vi "S4GUI_003.vi"(7 "Tab ObsEng":enum32{"Obs", "CCD modes", "Guider", "Eng"}(tab)) -> ()   [LabVIEW 2018] (continued)
        n2644 = call "Write GFOC.vi"("error in (no error)"=w5462, "Opt_Continuous.lvclass"=w5460, "Instrument in"=w5452) -> ("error out"=w5444:errorcluster, "Instrument out"=w5445:refnum<class "Instrument.lvclass">)  [unwired: 7 in]
        n2645 = call "Write Instrument.lvclass.vi"("error in (no error)"=w5444, "Instrument.lvclass"=w5445, "S4ACS_GUI in"=w5524) -> ("error out"=w5443:errorcluster, "S4ACS_GUI out"=w5442:refnum<class "S4GUI.lvclass">)  [unwired: 7 in]
      }
      event "Tab Acq Type": Value Change {
        # "Tab for choosing ACQUISITION MODE: Object, Test, Dflat, Sflat, Dark, Zero, Focus"
        n2646 = event-data() -> ("NewVal"=w5565:T1)  [unwired: 1 in]
        n2647 = case shown="\"ZERO\"" w5565 {
          tunnel: ["OBJECT" "OBJECT" "FLAT" "FLAT" "DARK" "ZERO" "FOCUS"] -> w5542
          tunnel: [w5634 w5639 w5647 w5652 w5657 w5662 w5667] -> w5541
          tunnel: [w5635 w5640 w5646 w5651 w5656 w5661 w5666] -> w5564
          tunnel: [w5636 w5641 w5645 w5650 w5655 w5660 w5665] -> w5538
          tunnel: [u32 0 u32 1 u32 2 u32 3 u32 4 u32 5 u32 6] -> w5533
          frame "OBJECT", Default {
            n2648 = local read "Object_obj"() -> (w5634:string)
            n2649 = local read "OBJECT Comments"() -> (w5636:string)
            n2650 = local read "object suffix"() -> (w5635:string)
          }
          frame "TEST" {
            n2651 = local read "TEST Comments"() -> (w5641:string)
            n2652 = local read "Object_test"() -> (w5639:string)
            n2653 = local read "test suffix"() -> (w5640:string)
          }
          frame "DFLAT" {
            n2654 = local read "DFLAT Comments"() -> (w5645:string)
            n2655 = local read "Object_dflat"() -> (w5647:string)
            n2656 = local read "dflat suffix"() -> (w5646:string)
          }
          frame "SFLAT" {
            n2657 = local read "SFLAT Comments"() -> (w5650:string)
            n2658 = local read "Object_sflat"() -> (w5652:string)
            n2659 = local read "sflat suffix"() -> (w5651:string)
          }
          frame "DARK" {
            n2660 = local read "Object_dark"() -> (w5657:string)
            n2661 = local read "dark suffix"() -> (w5656:string)
            n2662 = local read "DARK Comments"() -> (w5655:string)
          }
          frame "ZERO" {
            n2663 = local read "ZERO Comments"() -> (w5660:string)
            n2664 = local read "Object_zero"() -> (w5662:string)
            n2665 = local read "zero suffix"() -> (w5661:string)
          }
          frame "FOCUS" {
            n2666 = local read "FOCUS Comments"() -> (w5665:string)
            n2667 = local read "Object_focus"() -> (w5667:string)
            n2668 = local read "focus suffix"() -> (w5666:string)
          }
        }
        n2669 = local read "Observer"() -> (w5563:string)
        n2670 = call-dynamic "Write ExpMode.vi"("error in (no error)"=w5566, "ExpMode"=w5565, "S4GUI in"=w5567) -> ("error out"=w5559:errorcluster, "S4GUI out"=w5558:refnum<class "S4GUI.lvclass">)  [unwired: 7 in]
        n2671 = Concatenate Strings("ACQ TAB SELECTED:" ("User Event"), w5542) -> (w5560:string)
        n2672 = call-dynamic "Write User Event.vi"("error in (no error)"=w5559, "User Event"=w5560, "S4GUI in"=w5558) -> ("error out"=w5532:errorcluster, "S4GUI out"=w5531:refnum<class "S4GUI.lvclass">)  [unwired: 7 in]
        n2673 = call-dynamic "Write TabAcqType index.vi"("error in (no error)"=w5532, "TabAcqType index"=w5533, "S4GUI in"=w5531) -> ("error out"=w5528:errorcluster, "S4GUI out"=w5530:refnum<class "S4GUI.lvclass">)  [unwired: 7 in]
        n2674 = call-dynamic "Save TabAcqType index.vi"("error in (no error)"=w5528, "S4GUI in"=w5530) -> ("error out"=w5527:errorcluster, "S4GUI out"=w5529:refnum<class "S4GUI.lvclass">)  [unwired: 8 in]
        n2675 = call-dynamic "Read Publisher.lvclass.vi"("error in (no error)"=w5527, "S4GUI in"=w5529) -> ("error out"=w5556:errorcluster, "Publisher.lvclass"=w5552:refnum<class "Publisher.lvclass">, "S4GUI out"=w5557:refnum<class "S4GUI.lvclass">)  [unwired: 7 in]
        n2676 = call-dynamic "Write object.vi"("error in (no error)"=w5556, "object"=w5541, "Publisher in"=w5552) -> ("error out"=w5555:errorcluster, "Publisher out"=w5551:refnum<class "Publisher.lvclass">)  [unwired: 7 in]
        n2677 = call-dynamic "Write obstype.vi"("error in (no error)"=w5555, "obstype"=w5542, "Publisher in"=w5551) -> ("error out"=w5554:errorcluster, "Publisher out"=w5550:refnum<class "Publisher.lvclass">)  [unwired: 7 in]
        n2678 = call-dynamic "Write observer.vi"("error in (no error)"=w5554, "observer"=w5540, "Publisher in"=w5550) -> ("error out"=w5553:errorcluster, "Publisher out"=w5549:refnum<class "Publisher.lvclass">)  [unwired: 7 in]
        n2679 = call-dynamic "Write projid.vi"("error in (no error)"=w5553, "projid"=w5539, "Publisher in"=w5549) -> ("error out"=w5546:errorcluster, "Publisher out"=w5545:refnum<class "Publisher.lvclass">)  [unwired: 7 in]
        n2680 = call-dynamic "Write comments.vi"("error in (no error)"=w5546, "comments"=w5538, "Publisher in"=w5545) -> ("error out"=w5548:errorcluster, "Publisher out"=w5547:refnum<class "Publisher.lvclass">)  [unwired: 7 in]
        n2681 = call-dynamic "Write Publisher.lvclass.vi"("error in (no error)"=w5548, "Publisher.lvclass"=w5547, "S4GUI in"=w5557) -> ("error out"=w5544:errorcluster, "S4GUI out"=w5543:refnum<class "S4GUI.lvclass">)  [unwired: 7 in]
        n2682 = call-dynamic "Read AcquisitionA.vi"("error in (no error)"=w5544, "S4ACS_GUI in"=w5543) -> ("error out"=w5574:errorcluster, "Acquisition.lvclass"=w5575:refnum<class "Acquisition.lvclass">, "S4ACS_GUI out"=w5594:refnum<class "S4GUI.lvclass">)  [unwired: 7 in]
        n2683 = call-dynamic "Read AcquisitionC.vi"("error in (no error)"=w5532, "S4ACS_GUI in"=w5531) -> ("error out"=w5570:errorcluster, "Acquisition.lvclass"=w5571:refnum<class "Acquisition.lvclass">)  [unwired: 7 in, 1 out]
        n2684 = call "Read AcquisitionB.vi"("error in (no error)"=w5532, "S4ACS_GUI in"=w5531) -> ("error out"=w5572:errorcluster, "Acquisition.lvclass"=w5573:refnum<class "Acquisition.lvclass">)  [unwired: 7 in, 1 out]
        n2685 = call-dynamic "Read AcquisitionD.vi"("error in (no error)"=w5532, "S4ACS_GUI in"=w5531) -> ("error out"=w5568:errorcluster, "Acquisition.lvclass"=w5569:refnum<class "Acquisition.lvclass">)  [unwired: 7 in, 1 out]
        n2686 = To Lower Case(string=w5564) -> (all lower case string=w5562:string)
        n2687 = case shown="\"ZERO\"" w5565 {
          tunnel: [w5902 w6271 w6680] -> w5593
          tunnel: [w5901 w6270 w6679] -> w5592
          tunnel: [w5900 w6269 w6678] -> w5590
          tunnel: [w5899 w6268 w6677] -> w5589
          tunnel: [w5898 w6267 w6676] -> w5579
          tunnel: [w5897 w6266 w6675] -> w5578
          tunnel: [w5896 w6265 w6674] -> w5577
          tunnel: [w5895 w6264 w6673] -> w5576
          tunnel: w5575 -> [w5894 w6263 w6672]
          tunnel: w5574 -> [w5893 w6262 w6671]
          tunnel: w5573 -> [w5883 w6253 w6662]
          tunnel: w5572 -> [w5882 w6252 w6661]
          tunnel: w5571 -> [w5881 w6251 w6660]
          tunnel: w5570 -> [w5880 w6250 w6659]
          tunnel: w5569 -> [w5879 w6249 w6658]
          tunnel: w5568 -> [w5878 w6248 w6657]
          tunnel: w5541 -> [w5875 w6247 w6656]
          tunnel: w5538 -> [w5876 w6246 w6655]
          tunnel: w5563 -> [w5877 w6245 w6654]
          tunnel: w5562 -> [w5874 w6244 w6653]
          tunnel: w5542 -> [w5873 w6243 w6652]
          frame "ZERO" {
            w5892 = 1e-05 ("Exptime ch1")
            # "nome do arquivo .cfg"
            # "seção no arquivo .cfg"
            # "nome do arquivo .cfg"
            # "seção no arquivo .cfg"
            # "nome do arquivo .cfg"
            # "seção no arquivo .cfg"
            # "nome do arquivo .cfg"
            # "seção no arquivo .cfg"
            # "ZERO: EXPTIME=1E-5 (mandatory), shutter automatically closed, save current FRAME_TRANSFER (prev_FT) and reset FRAME_TRANSFER."
            n2688 = call "Read connection.vi"("error in (no error)"=w5880, "Server in"=w5881) -> ("error out"=w5886:errorcluster, "connection"=w5720:bool, "Server out"=w5887:refnum<class "Acquisition.lvclass">)  [unwired: 7 in]
            n2689 = call "Read connection.vi"("error in (no error)"=w5882, "Server in"=w5883) -> ("error out"=w5888:errorcluster, "connection"=w5771:bool, "Server out"=w5889:refnum<class "Acquisition.lvclass">)  [unwired: 7 in]
            n2690 = call "Read connection.vi"("error in (no error)"=w5893, "Server in"=w5894) -> ("error out"=w5890:errorcluster, "connection"=w5822:bool, "Server out"=w5891:refnum<class "Acquisition.lvclass">)  [unwired: 7 in]
            n2691 = call "Read connection.vi"("error in (no error)"=w5878, "Server in"=w5879) -> ("error out"=w5884:errorcluster, "connection"=w5669:bool, "Server out"=w5885:refnum<class "Acquisition.lvclass">)  [unwired: 7 in]
            n2692 = call-dynamic "Read Channel.vi"("error in (no error)"=w5888, "Acquisition in"=w5889) -> ("error out"=w5809:errorcluster, "Channel.lvclass"=w5808:refnum<class "Channel.lvclass">, "Acquisition out"=w5807:refnum<class "Acquisition.lvclass">)  [unwired: 7 in]
            n2693 = call-dynamic "Read Channel.vi"("error in (no error)"=w5884, "Acquisition in"=w5885) -> ("error out"=w5717:errorcluster, "Channel.lvclass"=w5718:refnum<class "Channel.lvclass">, "Acquisition out"=w5719:refnum<class "Acquisition.lvclass">)  [unwired: 7 in]
            n2694 = call-dynamic "Read Channel.vi"("error in (no error)"=w5886, "Acquisition in"=w5887) -> ("error out"=w5758:errorcluster, "Channel.lvclass"=w5757:refnum<class "Channel.lvclass">, "Acquisition out"=w5756:refnum<class "Acquisition.lvclass">)  [unwired: 7 in]
            n2695 = call-dynamic "Read Channel.vi"("error in (no error)"=w5890, "Acquisition in"=w5891) -> ("error out"=w5870:errorcluster, "Channel.lvclass"=w5871:refnum<class "Channel.lvclass">, "Acquisition out"=w5872:refnum<class "Acquisition.lvclass">)  [unwired: 7 in]
            n2696 = call-dynamic "Read Interface.vi"("error in (no error)"=w5717, "Channel in"=w5718) -> ("error out"=w5683:errorcluster, "Interface.lvclass"=w5682:refnum<class "Interface.lvclass">, "Channel out"=w5679:refnum<class "Channel.lvclass">)  [unwired: 7 in]
            n2697 = call-dynamic "Read Interface.vi"("error in (no error)"=w5809, "Channel in"=w5808) -> ("error out"=w5783:errorcluster, "Interface.lvclass"=w5784:refnum<class "Interface.lvclass">, "Channel out"=w5778:refnum<class "Channel.lvclass">)  [unwired: 7 in]
            n2698 = call-dynamic "Read Interface.vi"("error in (no error)"=w5758, "Channel in"=w5757) -> ("error out"=w5732:errorcluster, "Interface.lvclass"=w5733:refnum<class "Interface.lvclass">, "Channel out"=w5730:refnum<class "Channel.lvclass">)  [unwired: 7 in]
            n2699 = call-dynamic "Read Interface.vi"("error in (no error)"=w5870, "Channel in"=w5871) -> ("error out"=w5839:errorcluster, "Interface.lvclass"=w5840:refnum<class "Interface.lvclass">, "Channel out"=w5833:refnum<class "Channel.lvclass">)  [unwired: 7 in]
            n2700 = call-dynamic "Write restoreExpTime.vi"("error in (no error)"=w5683, "restoreExpTime"=TRUE, "Interface in"=w5682) -> ("error out"=w5676:errorcluster, "Interface out"=w5681:refnum<class "Interface.lvclass">)  [unwired: 7 in]
            n2701 = call-dynamic "Write restoreExpTime.vi"("error in (no error)"=w5783, "restoreExpTime"=TRUE, "Interface in"=w5784) -> ("error out"=w5780:errorcluster, "Interface out"=w5782:refnum<class "Interface.lvclass">)  [unwired: 7 in]
            n2702 = call-dynamic "Write restoreExpTime.vi"("error in (no error)"=w5732, "restoreExpTime"=TRUE, "Interface in"=w5733) -> ("error out"=w5725:errorcluster, "Interface out"=w5731:refnum<class "Interface.lvclass">)  [unwired: 7 in]
            n2703 = call-dynamic "Write restoreExpTime.vi"("error in (no error)"=w5839, "restoreExpTime"=TRUE, "Interface in"=w5840) -> ("error out"=w5829:errorcluster, "Interface out"=w5830:refnum<class "Interface.lvclass">)  [unwired: 7 in]
            n2704 = property on="Exptime ch1" class="DigNum (strict)"("Value"=w5892) -> ()  [unwired: 2 in, 2 out]
            n2705 = call-dynamic "Read target cluster.vi"("error in (no error)"=w5780, "Channel in"=w5778) -> ("error out"=w5779:errorcluster, "target cluster"=w5781:T31, "Channel out"=w5774:refnum<class "Channel.lvclass">)  [unwired: 7 in]
            n2706 = stacked-sequence {
              tunnel: [_ w5994] -> w5777
              tunnel: w5781 -> [_ w5993]
              tunnel: w5781 -> [w5991 _]
              tunnel: [w5990 _] -> w5786
              frame #0 {
                n2707 = Unbundle By Name(w5991) -> ("FRAME_TRANSFER"=w5990:bool)
              }
              frame #1 {
                # "closed"
                n2708 = Bundle By Name(cluster=w5993, "SHUTTER_MODE"=u8 2, "FRAME_TRANSFER"=FALSE) -> (w5994:T31)
              }
            }
            n2709 = call-dynamic "Read target cluster.vi"("error in (no error)"=w5676, "Channel in"=w5679) -> ("error out"=w5675:errorcluster, "target cluster"=w5677:T31, "Channel out"=w5678:refnum<class "Channel.lvclass">)  [unwired: 7 in]
            n2710 = stacked-sequence {
              tunnel: w5677 -> [_ w5933]
              tunnel: [_ w5932] -> w5673
              tunnel: w5677 -> [w5929 _]
              tunnel: [w5928 _] -> w5685
              frame #0 {
                n2711 = Unbundle By Name(w5929) -> ("FRAME_TRANSFER"=w5928:bool)
              }
              frame #1 {
                # "closed"
                n2712 = Bundle By Name(cluster=w5933, "SHUTTER_MODE"=u8 2, "FRAME_TRANSFER"=FALSE) -> (w5932:T31)
              }
            }
            n2713 = call-dynamic "Read target cluster.vi"("error in (no error)"=w5725, "Channel in"=w5730) -> ("error out"=w5724:errorcluster, "target cluster"=w5726:T31, "Channel out"=w5722:refnum<class "Channel.lvclass">)  [unwired: 7 in]
            n2714 = stacked-sequence {
              tunnel: [_ w5963] -> w5728
              tunnel: w5726 -> [_ w5962]
              tunnel: w5726 -> [w5960 _]
              tunnel: [w5959 _] -> w5735
              frame #0 {
                n2715 = Unbundle By Name(w5960) -> ("FRAME_TRANSFER"=w5959:bool)
              }
              frame #1 {
                # "closed"
                n2716 = Bundle By Name(cluster=w5962, "SHUTTER_MODE"=u8 2, "FRAME_TRANSFER"=FALSE) -> (w5963:T31)
              }
            }
            n2717 = property on="Exptime ch2" class="DigNum (strict)"("Value"=w5892) -> ()  [unwired: 2 in, 2 out]
            n2718 = call-dynamic "Read target cluster.vi"("error in (no error)"=w5829, "Channel in"=w5833) -> ("error out"=w5828:errorcluster, "target cluster"=w5831:T31, "Channel out"=w5832:refnum<class "Channel.lvclass">)  [unwired: 7 in]
            n2719 = stacked-sequence {
              tunnel: [_ w6026] -> w5837
              tunnel: w5831 -> [_ w6023]
              tunnel: w5831 -> [w6022 _]
              tunnel: [w6021 _] -> w5841
              frame #0 {
                n2720 = Unbundle By Name(w6022) -> ("FRAME_TRANSFER"=w6021:bool)
              }
              frame #1 {
                # "closed"
                n2721 = Bundle By Name(cluster=w6023, "SHUTTER_MODE"=u8 2, "FRAME_TRANSFER"=FALSE) -> (w6026:T31)
              }
            }
            n2722 = call-dynamic "Write PREV_FT.vi"("error in (no error)"=w5779, "PREV_FT"=w5786, "Interface in"=w5782) -> ("error out"=w5776:errorcluster, "Interface out"=w5772:refnum<class "Interface.lvclass">)  [unwired: 7 in]
            n2723 = call-dynamic "Write PREV_FT.vi"("error in (no error)"=w5675, "PREV_FT"=w5685, "Interface in"=w5681) -> ("error out"=w5674:errorcluster, "Interface out"=w5680:refnum<class "Interface.lvclass">)  [unwired: 7 in]
            n2724 = call-dynamic "Write PREV_FT.vi"("error in (no error)"=w5724, "PREV_FT"=w5735, "Interface in"=w5731) -> ("error out"=w5727:errorcluster, "Interface out"=w5729:refnum<class "Interface.lvclass">)  [unwired: 7 in]
            n2725 = property on="Exptime ch3" class="DigNum (strict)"("Value"=w5892) -> ()  [unwired: 2 in, 2 out]
            n2726 = call-dynamic "Write PREV_FT.vi"("error in (no error)"=w5828, "PREV_FT"=w5841, "Interface in"=w5830) -> ("error out"=w5834:errorcluster, "Interface out"=w5827:refnum<class "Interface.lvclass">)  [unwired: 7 in]
            n2727 = call-dynamic "Write target cluster.vi"("error in (no error)"=w5776, "target cluster"=w5777, "Channel in"=w5774) -> ("error out"=w5775:errorcluster, "Channel out"=w5773:refnum<class "Channel.lvclass">)  [unwired: 7 in]
            n2728 = call-dynamic "Write target cluster.vi"("error in (no error)"=w5674, "target cluster"=w5673, "Channel in"=w5678) -> ("error out"=w5672:errorcluster, "Channel out"=w5671:refnum<class "Channel.lvclass">)  [unwired: 7 in]
            n2729 = call-dynamic "Write target cluster.vi"("error in (no error)"=w5727, "target cluster"=w5728, "Channel in"=w5722) -> ("error out"=w5723:errorcluster, "Channel out"=w5721:refnum<class "Channel.lvclass">)  [unwired: 7 in]
            n2730 = call-dynamic "Write target cluster.vi"("error in (no error)"=w5834, "target cluster"=w5837, "Channel in"=w5832) -> ("error out"=w5836:errorcluster, "Channel out"=w5835:refnum<class "Channel.lvclass">)  [unwired: 7 in]
            n2731 = Flatten To String(anything=w5777, error in (no error)=w5775) -> (data string=w5810:string, error out=w5811:errorcluster)  [unwired: 2 in, 1 out]
            n2732 = Flatten To String(anything=w5673, error in (no error)=w5672) -> (data string=w5716:string, error out=w5715:errorcluster)  [unwired: 2 in, 1 out]
            n2733 = Flatten To String(anything=w5728, error in (no error)=w5723) -> (data string=w5759:string, error out=w5760:errorcluster)  [unwired: 2 in, 1 out]
            n2734 = Flatten To String(anything=w5837, error in (no error)=w5836) -> (data string=w5869:string, error out=w5868:errorcluster)  [unwired: 2 in, 1 out]
            n2735 = property on="Exptime ch4" class="DigNum (strict)"("Value"=w5892) -> ()  [unwired: 2 in, 2 out]
            n2736 = call "Write flatted cluster.vi"("error in (no error)"=w5811, "flatted cluster"=w5810, "Interface in"=w5772) -> ("error out"=w5813:errorcluster, "Interface out"=w5812:refnum<class "Interface.lvclass">)  [unwired: 7 in]
            n2737 = call "Write flatted cluster.vi"("error in (no error)"=w5715, "flatted cluster"=w5716, "Interface in"=w5680) -> ("error out"=w5713:errorcluster, "Interface out"=w5714:refnum<class "Interface.lvclass">)  [unwired: 7 in]
            n2738 = call "Write flatted cluster.vi"("error in (no error)"=w5760, "flatted cluster"=w5759, "Interface in"=w5729) -> ("error out"=w5762:errorcluster, "Interface out"=w5761:refnum<class "Interface.lvclass">)  [unwired: 7 in]
            n2739 = call "Write flatted cluster.vi"("error in (no error)"=w5868, "flatted cluster"=w5869, "Interface in"=w5827) -> ("error out"=w5866:errorcluster, "Interface out"=w5867:refnum<class "Interface.lvclass">)  [unwired: 7 in]
            n2740 = call-dynamic "Write Interface.vi"("error in (no error)"=w5813, "Interface.lvclass"=w5812, "Channel in"=w5773) -> ("error out"=w5815:errorcluster, "Channel out"=w5816:refnum<class "Channel.lvclass">)  [unwired: 7 in]
            n2741 = call-dynamic "Write Interface.vi"("error in (no error)"=w5713, "Interface.lvclass"=w5714, "Channel in"=w5671) -> ("error out"=w5711:errorcluster, "Channel out"=w5710:refnum<class "Channel.lvclass">)  [unwired: 7 in]
            n2742 = call-dynamic "Write Interface.vi"("error in (no error)"=w5762, "Interface.lvclass"=w5761, "Channel in"=w5721) -> ("error out"=w5764:errorcluster, "Channel out"=w5765:refnum<class "Channel.lvclass">)  [unwired: 7 in]
            n2743 = call-dynamic "Write Interface.vi"("error in (no error)"=w5866, "Interface.lvclass"=w5867, "Channel in"=w5835) -> ("error out"=w5864:errorcluster, "Channel out"=w5863:refnum<class "Channel.lvclass">)  [unwired: 7 in]
            n2744 = call "Write section_name.vi"("error in (no error)"=w5815, "section_name"="CCD_ACS2", "Channel in"=w5816) -> ("error out"=w5814:errorcluster, "Channel out"=w5819:refnum<class "Channel.lvclass">)  [unwired: 7 in]
            n2745 = call "Write section_name.vi"("error in (no error)"=w5711, "section_name"="CCD_ACS4", "Channel in"=w5710) -> ("error out"=w5712:errorcluster, "Channel out"=w5707:refnum<class "Channel.lvclass">)  [unwired: 7 in]
            n2746 = call "Write section_name.vi"("error in (no error)"=w5764, "section_name"="CCD_ACS3", "Channel in"=w5765) -> ("error out"=w5763:errorcluster, "Channel out"=w5768:refnum<class "Channel.lvclass">)  [unwired: 7 in]
            n2747 = call "Write section_name.vi"("error in (no error)"=w5864, "section_name"="CCD_ACS1", "Channel in"=w5863) -> ("error out"=w5865:errorcluster, "Channel out"=w5860:refnum<class "Channel.lvclass">)  [unwired: 7 in]
            n2748 = call-dynamic "save config.vi"("error in (no error)"=w5814, "file config"="lastsaved.cfg", "Channel in"=w5819) -> ("error out"=w5789:errorcluster, "Channel out"=w5790:refnum<class "Channel.lvclass">)  [unwired: 7 in]
            n2749 = call-dynamic "save config.vi"("error in (no error)"=w5712, "file config"="lastsaved.cfg", "Channel in"=w5707) -> ("error out"=w5688:errorcluster, "Channel out"=w5689:refnum<class "Channel.lvclass">)  [unwired: 7 in]
            n2750 = call-dynamic "save config.vi"("error in (no error)"=w5763, "file config"="lastsaved.cfg", "Channel in"=w5768) -> ("error out"=w5737:errorcluster, "Channel out"=w5739:refnum<class "Channel.lvclass">)  [unwired: 7 in]
            n2751 = call-dynamic "save config.vi"("error in (no error)"=w5865, "file config"="lastsaved.cfg", "Channel in"=w5860) -> ("error out"=w5850:errorcluster, "Channel out"=w5851:refnum<class "Channel.lvclass">)  [unwired: 7 in]
            n2752 = local read "Filter2"() -> (w5791:u8)
            n2753 = local read "Filter4"() -> (w5705:u8)
            n2754 = local read "Filter3"() -> (w5755:u8)
            n2755 = local read "Filter1"() -> (w5852:u8)
            n2756 = call-dynamic "Write Filter.vi"("error in (no error)"=w5789, "Filter"=w5791, "Channel in"=w5790) -> ("error out"=w5798:errorcluster, "Channel out"=w5799:refnum<class "Channel.lvclass">)  [unwired: 7 in]
            n2757 = call-dynamic "Write Filter.vi"("error in (no error)"=w5688, "Filter"=w5705, "Channel in"=w5689) -> ("error out"=w5698:errorcluster, "Channel out"=w5697:refnum<class "Channel.lvclass">)  [unwired: 7 in]
            n2758 = call-dynamic "Write Filter.vi"("error in (no error)"=w5737, "Filter"=w5755, "Channel in"=w5739) -> ("error out"=w5748:errorcluster, "Channel out"=w5747:refnum<class "Channel.lvclass">)  [unwired: 7 in]
            n2759 = call-dynamic "Write Filter.vi"("error in (no error)"=w5850, "Filter"=w5852, "Channel in"=w5851) -> ("error out"=w5859:errorcluster, "Channel out"=w5849:refnum<class "Channel.lvclass">)  [unwired: 7 in]
            n2760 = call-dynamic "Read Interface.vi"("error in (no error)"=w5798, "Channel in"=w5799) -> ("error out"=w5796:errorcluster, "Interface.lvclass"=w5801:refnum<class "Interface.lvclass">, "Channel out"=w5800:refnum<class "Channel.lvclass">)  [unwired: 7 in]
            n2761 = call-dynamic "Read Interface.vi"("error in (no error)"=w5698, "Channel in"=w5697) -> ("error out"=w5700:errorcluster, "Interface.lvclass"=w5695:refnum<class "Interface.lvclass">, "Channel out"=w5696:refnum<class "Channel.lvclass">)  [unwired: 7 in]
            n2762 = call-dynamic "Read Interface.vi"("error in (no error)"=w5748, "Channel in"=w5747) -> ("error out"=w5750:errorcluster, "Interface.lvclass"=w5745:refnum<class "Interface.lvclass">, "Channel out"=w5746:refnum<class "Channel.lvclass">)  [unwired: 7 in]
            n2763 = call-dynamic "Read Interface.vi"("error in (no error)"=w5859, "Channel in"=w5849) -> ("error out"=w5857:errorcluster, "Interface.lvclass"=w5848:refnum<class "Interface.lvclass">, "Channel out"=w5842:refnum<class "Channel.lvclass">)  [unwired: 7 in]
            n2764 = call-dynamic "Write Suffix.vi"("error in (no error)"=w5796, "Suffix"=w5874, "Interface in"=w5801) -> ("error out"=w5792:errorcluster, "Interface out"=w5802:refnum<class "Interface.lvclass">)  [unwired: 7 in]
            n2765 = call-dynamic "Write Suffix.vi"("error in (no error)"=w5700, "Suffix"=w5874, "Interface in"=w5695) -> ("error out"=w5704:errorcluster, "Interface out"=w5694:refnum<class "Interface.lvclass">)  [unwired: 7 in]
            n2766 = call-dynamic "Write Suffix.vi"("error in (no error)"=w5750, "Suffix"=w5874, "Interface in"=w5745) -> ("error out"=w5754:errorcluster, "Interface out"=w5744:refnum<class "Interface.lvclass">)  [unwired: 7 in]
            n2767 = call-dynamic "Write Suffix.vi"("error in (no error)"=w5857, "Suffix"=w5874, "Interface in"=w5848) -> ("error out"=w5853:errorcluster, "Interface out"=w5847:refnum<class "Interface.lvclass">)  [unwired: 7 in]
            n2768 = call-dynamic "Write ObsType.vi"("error in (no error)"=w5792, "ObsType"=w5873, "Interface in"=w5802) -> ("error out"=w5793:errorcluster, "Interface out"=w5803:refnum<class "Interface.lvclass">)  [unwired: 7 in]
            n2769 = call-dynamic "Write ObsType.vi"("error in (no error)"=w5704, "ObsType"=w5873, "Interface in"=w5694) -> ("error out"=w5703:errorcluster, "Interface out"=w5693:refnum<class "Interface.lvclass">)  [unwired: 7 in]
            n2770 = call-dynamic "Write ObsType.vi"("error in (no error)"=w5754, "ObsType"=w5873, "Interface in"=w5744) -> ("error out"=w5753:errorcluster, "Interface out"=w5743:refnum<class "Interface.lvclass">)  [unwired: 7 in]
            n2771 = call-dynamic "Write ObsType.vi"("error in (no error)"=w5853, "ObsType"=w5873, "Interface in"=w5847) -> ("error out"=w5854:errorcluster, "Interface out"=w5846:refnum<class "Interface.lvclass">)  [unwired: 7 in]
            n2772 = call-dynamic "Write Object.vi"("error in (no error)"=w5793, "Object"=w5875, "Interface in"=w5803) -> ("error out"=w5794:errorcluster, "Interface out"=w5804:refnum<class "Interface.lvclass">)  [unwired: 7 in]
            n2773 = call-dynamic "Write Object.vi"("error in (no error)"=w5703, "Object"=w5875, "Interface in"=w5693) -> ("error out"=w5702:errorcluster, "Interface out"=w5692:refnum<class "Interface.lvclass">)  [unwired: 7 in]
            n2774 = call-dynamic "Write Object.vi"("error in (no error)"=w5753, "Object"=w5875, "Interface in"=w5743) -> ("error out"=w5752:errorcluster, "Interface out"=w5742:refnum<class "Interface.lvclass">)  [unwired: 7 in]
            n2775 = call-dynamic "Write Object.vi"("error in (no error)"=w5854, "Object"=w5875, "Interface in"=w5846) -> ("error out"=w5855:errorcluster, "Interface out"=w5845:refnum<class "Interface.lvclass">)  [unwired: 7 in]
            n2776 = call-dynamic "Write Comments.vi"("error in (no error)"=w5794, "Comments"=w5876, "Interface in"=w5804) -> ("error out"=w5795:errorcluster, "Interface out"=w5805:refnum<class "Interface.lvclass">)  [unwired: 7 in]
            n2777 = call-dynamic "Write Comments.vi"("error in (no error)"=w5702, "Comments"=w5876, "Interface in"=w5692) -> ("error out"=w5701:errorcluster, "Interface out"=w5691:refnum<class "Interface.lvclass">)  [unwired: 7 in]
            n2778 = call-dynamic "Write Comments.vi"("error in (no error)"=w5752, "Comments"=w5876, "Interface in"=w5742) -> ("error out"=w5751:errorcluster, "Interface out"=w5741:refnum<class "Interface.lvclass">)  [unwired: 7 in]
            n2779 = call-dynamic "Write Comments.vi"("error in (no error)"=w5855, "Comments"=w5876, "Interface in"=w5845) -> ("error out"=w5856:errorcluster, "Interface out"=w5844:refnum<class "Interface.lvclass">)  [unwired: 7 in]
            n2780 = call-dynamic "Write Observer.vi"("error in (no error)"=w5701, "Observer"=w5877, "Interface in"=w5691) -> ("error out"=w5699:errorcluster, "Interface out"=w5690:refnum<class "Interface.lvclass">)  [unwired: 7 in]
            n2781 = call-dynamic "Write Observer.vi"("error in (no error)"=w5751, "Observer"=w5877, "Interface in"=w5741) -> ("error out"=w5749:errorcluster, "Interface out"=w5740:refnum<class "Interface.lvclass">)  [unwired: 7 in]
            n2782 = call-dynamic "Write Observer.vi"("error in (no error)"=w5795, "Observer"=w5877, "Interface in"=w5805) -> ("error out"=w5797:errorcluster, "Interface out"=w5806:refnum<class "Interface.lvclass">)  [unwired: 7 in]
            n2783 = call-dynamic "Write Observer.vi"("error in (no error)"=w5856, "Observer"=w5877, "Interface in"=w5844) -> ("error out"=w5858:errorcluster, "Interface out"=w5843:refnum<class "Interface.lvclass">)  [unwired: 7 in]
            n2784 = call-dynamic "Write Interface.vi"("error in (no error)"=w5699, "Interface.lvclass"=w5690, "Channel in"=w5696) -> ("error out"=w5687:errorcluster, "Channel out"=w5686:refnum<class "Channel.lvclass">)  [unwired: 7 in]
            n2785 = call-dynamic "Write Interface.vi"("error in (no error)"=w5749, "Interface.lvclass"=w5740, "Channel in"=w5746) -> ("error out"=w5736:errorcluster, "Channel out"=w5738:refnum<class "Channel.lvclass">)  [unwired: 7 in]
            n2786 = call-dynamic "Write Interface.vi"("error in (no error)"=w5858, "Interface.lvclass"=w5843, "Channel in"=w5842) -> ("error out"=w5825:errorcluster, "Channel out"=w5826:refnum<class "Channel.lvclass">)  [unwired: 7 in]
            n2787 = call-dynamic "Write Interface.vi"("error in (no error)"=w5797, "Interface.lvclass"=w5806, "Channel in"=w5800) -> ("error out"=w5788:errorcluster, "Channel out"=w5787:refnum<class "Channel.lvclass">)  [unwired: 7 in]
            n2788 = case shown="True" w5822 {
              tunnel: w5826 -> [w5997 w6001]
              tunnel: w5825 -> [w5996 w6000]
              tunnel: [w5997 w5999] -> w5824
              tunnel: [w5996 w5998] -> w5823
              frame False {
              }
              frame True {
                n2789 = call-dynamic "Read State Machine.vi"("error in (no error)"=w6000, "Device in"=w6001) -> ("error out"=w6003:errorcluster, "State Machine.lvclass"=w6006:refnum<class "State Machine.lvclass">, "Device out"=w6018:refnum<class "Channel.lvclass">)  [unwired: 7 in]
                n2790 = call-dynamic "Read ref StatesQueue.vi"("error in (no error)"=w6003, "State Machine in"=w6006) -> ("error out"=w6010:errorcluster, "ref StatesQueue"=w6009:refnum<queue>, "State Machine out"=w6005:refnum<class "State Machine.lvclass">)  [unwired: 7 in]
                n2791 = Flush Queue(queue=w6009, error in (no error)=w6010) -> (queue out=w6011:refnum<queue>, error out=w6015:errorcluster)  [unwired: 1 out]
                n2792 = Enqueue Element(queue=w6011, element=u32 300 ("State"), error in (no error)=w6015) -> (queue out=w6012:refnum<queue>, error out=w6016:errorcluster)  [unwired: 1 in, 1 out]
                n2793 = Enqueue Element(queue=w6012, element=u32 60 ("State"), error in (no error)=w6016) -> (queue out=w6013:refnum<queue>, error out=w6014:errorcluster)  [unwired: 1 in, 1 out]
                n2794 = call-dynamic "Write ref StatesQueue.vi"("error in (no error)"=w6014, "ref StatesQueue"=w6013, "State Machine in"=w6005) -> ("error out"=w6002:errorcluster, "State Machine out"=w6004:refnum<class "State Machine.lvclass">)  [unwired: 7 in]
                n2795 = call-dynamic "Write State.vi"("error in (no error)"=w6002, "State"=0, "State Machine in"=w6004) -> ("error out"=w6020:errorcluster, "State Machine out"=w6017:refnum<class "State Machine.lvclass">)  [unwired: 7 in]
                n2796 = call-dynamic "Write State Machine.vi"("error in (no error)"=w6020, "State Machine.lvclass"=w6017, "Device in"=w6018) -> ("error out"=w5998:errorcluster, "Device out"=w5999:refnum<class "Channel.lvclass">)  [unwired: 7 in]
              }
            }
            n2797 = case shown="True" w5771 {
              tunnel: [w5965 w5989] -> w5821
              tunnel: [w5966 w5988] -> w5820
              tunnel: w5788 -> [w5965 w5983]
              tunnel: w5787 -> [w5966 w5982]
              frame False {
              }
              frame True {
                n2798 = call-dynamic "Read State Machine.vi"("error in (no error)"=w5983, "Device in"=w5982) -> ("error out"=w5968:errorcluster, "State Machine.lvclass"=w5970:refnum<class "State Machine.lvclass">, "Device out"=w5986:refnum<class "Channel.lvclass">)  [unwired: 7 in]
                n2799 = call-dynamic "Read ref StatesQueue.vi"("error in (no error)"=w5968, "State Machine in"=w5970) -> ("error out"=w5975:errorcluster, "ref StatesQueue"=w5974:refnum<queue>, "State Machine out"=w5971:refnum<class "State Machine.lvclass">)  [unwired: 7 in]
                n2800 = Flush Queue(queue=w5974, error in (no error)=w5975) -> (queue out=w5976:refnum<queue>, error out=w5980:errorcluster)  [unwired: 1 out]
                n2801 = Enqueue Element(queue=w5976, element=u32 300 ("State"), error in (no error)=w5980) -> (queue out=w5977:refnum<queue>, error out=w5981:errorcluster)  [unwired: 1 in, 1 out]
                n2802 = Enqueue Element(queue=w5977, element=u32 60 ("State"), error in (no error)=w5981) -> (queue out=w5978:refnum<queue>, error out=w5979:errorcluster)  [unwired: 1 in, 1 out]
                n2803 = call-dynamic "Write ref StatesQueue.vi"("error in (no error)"=w5979, "ref StatesQueue"=w5978, "State Machine in"=w5971) -> ("error out"=w5967:errorcluster, "State Machine out"=w5969:refnum<class "State Machine.lvclass">)  [unwired: 7 in]
                n2804 = call-dynamic "Write State.vi"("error in (no error)"=w5967, "State"=0, "State Machine in"=w5969) -> ("error out"=w5984:errorcluster, "State Machine out"=w5987:refnum<class "State Machine.lvclass">)  [unwired: 7 in]
                n2805 = call-dynamic "Write State Machine.vi"("error in (no error)"=w5984, "State Machine.lvclass"=w5987, "Device in"=w5986) -> ("error out"=w5989:errorcluster, "Device out"=w5988:refnum<class "Channel.lvclass">)  [unwired: 7 in]
              }
            }
            n2806 = case shown="True" w5720 {
              tunnel: [w5935 w5958] -> w5770
              tunnel: [w5934 w5957] -> w5769
              tunnel: w5738 -> [w5934 w5952]
              tunnel: w5736 -> [w5935 w5951]
              frame False {
              }
              frame True {
                n2807 = call-dynamic "Read State Machine.vi"("error in (no error)"=w5951, "Device in"=w5952) -> ("error out"=w5937:errorcluster, "State Machine.lvclass"=w5939:refnum<class "State Machine.lvclass">, "Device out"=w5955:refnum<class "Channel.lvclass">)  [unwired: 7 in]
                n2808 = call-dynamic "Read ref StatesQueue.vi"("error in (no error)"=w5937, "State Machine in"=w5939) -> ("error out"=w5944:errorcluster, "ref StatesQueue"=w5943:refnum<queue>, "State Machine out"=w5940:refnum<class "State Machine.lvclass">)  [unwired: 7 in]
                n2809 = Flush Queue(queue=w5943, error in (no error)=w5944) -> (queue out=w5945:refnum<queue>, error out=w5949:errorcluster)  [unwired: 1 out]
                n2810 = Enqueue Element(queue=w5945, element=u32 300 ("State"), error in (no error)=w5949) -> (queue out=w5946:refnum<queue>, error out=w5950:errorcluster)  [unwired: 1 in, 1 out]
                n2811 = Enqueue Element(queue=w5946, element=u32 60 ("State"), error in (no error)=w5950) -> (queue out=w5947:refnum<queue>, error out=w5948:errorcluster)  [unwired: 1 in, 1 out]
                n2812 = call-dynamic "Write ref StatesQueue.vi"("error in (no error)"=w5948, "ref StatesQueue"=w5947, "State Machine in"=w5940) -> ("error out"=w5936:errorcluster, "State Machine out"=w5938:refnum<class "State Machine.lvclass">)  [unwired: 7 in]
                n2813 = call-dynamic "Write State.vi"("error in (no error)"=w5936, "State"=0, "State Machine in"=w5938) -> ("error out"=w5953:errorcluster, "State Machine out"=w5956:refnum<class "State Machine.lvclass">)  [unwired: 7 in]
                n2814 = call-dynamic "Write State Machine.vi"("error in (no error)"=w5953, "State Machine.lvclass"=w5956, "Device in"=w5955) -> ("error out"=w5958:errorcluster, "Device out"=w5957:refnum<class "Channel.lvclass">)  [unwired: 7 in]
              }
            }
            n2815 = case shown="True" w5669 {
              tunnel: [w5903 w5923] -> w5706
              tunnel: w5687 -> [w5903 w5922]
              tunnel: w5686 -> [w5904 w5921]
              tunnel: [w5904 w5905] -> w5670
              frame False {
              }
              frame True {
                n2816 = call-dynamic "Read State Machine.vi"("error in (no error)"=w5922, "Device in"=w5921) -> ("error out"=w5908:errorcluster, "State Machine.lvclass"=w5909:refnum<class "State Machine.lvclass">, "Device out"=w5925:refnum<class "Channel.lvclass">)  [unwired: 7 in]
                n2817 = call-dynamic "Read ref StatesQueue.vi"("error in (no error)"=w5908, "State Machine in"=w5909) -> ("error out"=w5914:errorcluster, "ref StatesQueue"=w5913:refnum<queue>, "State Machine out"=w5910:refnum<class "State Machine.lvclass">)  [unwired: 7 in]
                n2818 = Flush Queue(queue=w5913, error in (no error)=w5914) -> (queue out=w5915:refnum<queue>, error out=w5919:errorcluster)  [unwired: 1 out]
                n2819 = Enqueue Element(queue=w5915, element=u32 300 ("State"), error in (no error)=w5919) -> (queue out=w5916:refnum<queue>, error out=w5920:errorcluster)  [unwired: 1 in, 1 out]
                n2820 = Enqueue Element(queue=w5916, element=u32 60 ("State"), error in (no error)=w5920) -> (queue out=w5917:refnum<queue>, error out=w5918:errorcluster)  [unwired: 1 in, 1 out]
                n2821 = call-dynamic "Write ref StatesQueue.vi"("error in (no error)"=w5918, "ref StatesQueue"=w5917, "State Machine in"=w5910) -> ("error out"=w5907:errorcluster, "State Machine out"=w5906:refnum<class "State Machine.lvclass">)  [unwired: 7 in]
                n2822 = call-dynamic "Write State.vi"("error in (no error)"=w5907, "State"=0, "State Machine in"=w5906) -> ("error out"=w5927:errorcluster, "State Machine out"=w5924:refnum<class "State Machine.lvclass">)  [unwired: 7 in]
                n2823 = call-dynamic "Write State Machine.vi"("error in (no error)"=w5927, "State Machine.lvclass"=w5924, "Device in"=w5925) -> ("error out"=w5923:errorcluster, "Device out"=w5905:refnum<class "Channel.lvclass">)  [unwired: 7 in]
              }
            }
            n2824 = call-dynamic "Write Channel.vi"("error in (no error)"=w5821, "Channel.lvclass"=w5820, "Acquisition in"=w5807) -> ("error out"=w5899:errorcluster, "Acquisition out"=w5900:refnum<class "Acquisition.lvclass">)  [unwired: 7 in]
            n2825 = call-dynamic "Write Channel.vi"("error in (no error)"=w5823, "Channel.lvclass"=w5824, "Acquisition in"=w5872) -> ("error out"=w5901:errorcluster, "Acquisition out"=w5902:refnum<class "Acquisition.lvclass">)  [unwired: 7 in]
            n2826 = call-dynamic "Write Channel.vi"("error in (no error)"=w5770, "Channel.lvclass"=w5769, "Acquisition in"=w5756) -> ("error out"=w5897:errorcluster, "Acquisition out"=w5898:refnum<class "Acquisition.lvclass">)  [unwired: 7 in]
            n2827 = call-dynamic "Write Channel.vi"("error in (no error)"=w5706, "Channel.lvclass"=w5670, "Acquisition in"=w5719) -> ("error out"=w5895:errorcluster, "Acquisition out"=w5896:refnum<class "Acquisition.lvclass">)  [unwired: 7 in]
          }
          frame "DARK" {
            # "nome do arquivo .cfg"
            # "seção no arquivo .cfg"
            # "closed"
            # "nome do arquivo .cfg"
            # "seção no arquivo .cfg"
            # "closed"
            # "nome do arquivo .cfg"
            # "seção no arquivo .cfg"
            # "closed"
            # "nome do arquivo .cfg"
            # "seção no arquivo .cfg"
            # "closed"
            # "DARK: Shutter automatically closed and restore FRAME_TRANSFER."
            n2828 = call "Read connection.vi"("error in (no error)"=w6248, "Server in"=w6249) -> ("error out"=w6254:errorcluster, "connection"=w6027:bool, "Server out"=w6255:refnum<class "Acquisition.lvclass">)  [unwired: 7 in]
            n2829 = call "Read connection.vi"("error in (no error)"=w6250, "Server in"=w6251) -> ("error out"=w6256:errorcluster, "connection"=w6028:bool, "Server out"=w6257:refnum<class "Acquisition.lvclass">)  [unwired: 7 in]
            n2830 = call "Read connection.vi"("error in (no error)"=w6252, "Server in"=w6253) -> ("error out"=w6258:errorcluster, "connection"=w6029:bool, "Server out"=w6259:refnum<class "Acquisition.lvclass">)  [unwired: 7 in]
            n2831 = call "Read connection.vi"("error in (no error)"=w6262, "Server in"=w6263) -> ("error out"=w6260:errorcluster, "connection"=w6030:bool, "Server out"=w6261:refnum<class "Acquisition.lvclass">)  [unwired: 7 in]
            n2832 = call-dynamic "Read Channel.vi"("error in (no error)"=w6254, "Acquisition in"=w6255) -> ("error out"=w6081:errorcluster, "Channel.lvclass"=w6082:refnum<class "Channel.lvclass">, "Acquisition out"=w6083:refnum<class "Acquisition.lvclass">)  [unwired: 7 in]
            n2833 = call-dynamic "Read Channel.vi"("error in (no error)"=w6256, "Acquisition in"=w6257) -> ("error out"=w6123:errorcluster, "Channel.lvclass"=w6122:refnum<class "Channel.lvclass">, "Acquisition out"=w6121:refnum<class "Acquisition.lvclass">)  [unwired: 7 in]
            n2834 = call-dynamic "Read Channel.vi"("error in (no error)"=w6258, "Acquisition in"=w6259) -> ("error out"=w6176:errorcluster, "Channel.lvclass"=w6175:refnum<class "Channel.lvclass">, "Acquisition out"=w6174:refnum<class "Acquisition.lvclass">)  [unwired: 7 in]
            n2835 = call-dynamic "Read Channel.vi"("error in (no error)"=w6260, "Acquisition in"=w6261) -> ("error out"=w6240:errorcluster, "Channel.lvclass"=w6241:refnum<class "Channel.lvclass">, "Acquisition out"=w6242:refnum<class "Acquisition.lvclass">)  [unwired: 7 in]
            n2836 = call-dynamic "Read Interface.vi"("error in (no error)"=w6081, "Channel in"=w6082) -> ("error out"=w6044:errorcluster, "Interface.lvclass"=w6043:refnum<class "Interface.lvclass">, "Channel out"=w6039:refnum<class "Channel.lvclass">)  [unwired: 7 in]
            n2837 = call-dynamic "Read Interface.vi"("error in (no error)"=w6123, "Channel in"=w6122) -> ("error out"=w6095:errorcluster, "Interface.lvclass"=w6097:refnum<class "Interface.lvclass">, "Channel out"=w6092:refnum<class "Channel.lvclass">)  [unwired: 7 in]
            n2838 = call-dynamic "Read Interface.vi"("error in (no error)"=w6176, "Channel in"=w6175) -> ("error out"=w6150:errorcluster, "Interface.lvclass"=w6149:refnum<class "Interface.lvclass">, "Channel out"=w6145:refnum<class "Channel.lvclass">)  [unwired: 7 in]
            n2839 = call-dynamic "Read Interface.vi"("error in (no error)"=w6240, "Channel in"=w6241) -> ("error out"=w6202:errorcluster, "Interface.lvclass"=w6203:refnum<class "Interface.lvclass">, "Channel out"=w6198:refnum<class "Channel.lvclass">)  [unwired: 7 in]
            n2840 = call-dynamic "Read restoreExpTime.vi"("error in (no error)"=w6044, "Interface in"=w6043) -> ("error out"=w6041:errorcluster, "restoreExpTime"=w6040:bool, "Interface out"=w6042:refnum<class "Interface.lvclass">)  [unwired: 7 in]
            n2841 = call-dynamic "Read restoreExpTime.vi"("error in (no error)"=w6095, "Interface in"=w6097) -> ("error out"=w6094:errorcluster, "restoreExpTime"=w6093:bool, "Interface out"=w6096:refnum<class "Interface.lvclass">)  [unwired: 7 in]
            n2842 = call-dynamic "Read restoreExpTime.vi"("error in (no error)"=w6150, "Interface in"=w6149) -> ("error out"=w6147:errorcluster, "restoreExpTime"=w6146:bool, "Interface out"=w6148:refnum<class "Interface.lvclass">)  [unwired: 7 in]
            n2843 = call-dynamic "Read restoreExpTime.vi"("error in (no error)"=w6202, "Interface in"=w6203) -> ("error out"=w6200:errorcluster, "restoreExpTime"=w6199:bool, "Interface out"=w6201:refnum<class "Interface.lvclass">)  [unwired: 7 in]
            n2844 = case shown="True" w6040 {
              tunnel: w6042 -> [w6385 w6396]
              tunnel: w6041 -> [w6384 w6394]
              tunnel: [w6384 w6387] -> w6046
              tunnel: [w6385 w6386] -> w6045
              frame False {
              }
              frame True {
                n2845 = call-dynamic "Write restoreExpTime.vi"("error in (no error)"=w6394, "restoreExpTime"=FALSE, "Interface in"=w6396) -> ("error out"=w6392:errorcluster, "Interface out"=w6395:refnum<class "Interface.lvclass">)  [unwired: 7 in]
                n2846 = call-dynamic "Read prev ExpTime.vi"("error in (no error)"=w6392, "Interface in"=w6395) -> ("error out"=w6389:errorcluster, "prev ExpTime"=w6390:dbl, "Interface out"=w6391:refnum<class "Interface.lvclass">)  [unwired: 7 in]
                n2847 = property on="Exptime ch4" class="DigNum (strict)"(error in=w6389, "Value"=w6390) -> (error out=w6388:errorcluster)  [unwired: 1 in, 1 out]
                n2848 = call "Write Exposure Time.vi"("error in (no error)"=w6388, "Exposure Time"=w6390, "Interface in"=w6391) -> ("error out"=w6387:errorcluster, "Interface out"=w6386:refnum<class "Interface.lvclass">)  [unwired: 7 in]
              }
            }
            n2849 = case shown="True" w6093 {
              tunnel: w6096 -> [w6398 w6409]
              tunnel: [w6398 w6399] -> w6099
              tunnel: w6094 -> [w6397 w6408]
              tunnel: [w6397 w6400] -> w6098
              frame False {
              }
              frame True {
                n2850 = call-dynamic "Write restoreExpTime.vi"("error in (no error)"=w6408, "restoreExpTime"=FALSE, "Interface in"=w6409) -> ("error out"=w6405:errorcluster, "Interface out"=w6406:refnum<class "Interface.lvclass">)  [unwired: 7 in]
                n2851 = call-dynamic "Read prev ExpTime.vi"("error in (no error)"=w6405, "Interface in"=w6406) -> ("error out"=w6402:errorcluster, "prev ExpTime"=w6403:dbl, "Interface out"=w6404:refnum<class "Interface.lvclass">)  [unwired: 7 in]
                n2852 = property on="Exptime ch3" class="DigNum (strict)"(error in=w6402, "Value"=w6403) -> (error out=w6401:errorcluster)  [unwired: 1 in, 1 out]
                n2853 = call "Write Exposure Time.vi"("error in (no error)"=w6401, "Exposure Time"=w6403, "Interface in"=w6404) -> ("error out"=w6400:errorcluster, "Interface out"=w6399:refnum<class "Interface.lvclass">)  [unwired: 7 in]
              }
            }
            n2854 = case shown="True" w6146 {
              tunnel: w6148 -> [w6411 w6422]
              tunnel: [w6411 w6412] -> w6152
              tunnel: w6147 -> [w6410 w6420]
              tunnel: [w6410 w6413] -> w6151
              frame False {
              }
              frame True {
                n2855 = call-dynamic "Write restoreExpTime.vi"("error in (no error)"=w6420, "restoreExpTime"=FALSE, "Interface in"=w6422) -> ("error out"=w6419:errorcluster, "Interface out"=w6421:refnum<class "Interface.lvclass">)  [unwired: 7 in]
                n2856 = call-dynamic "Read prev ExpTime.vi"("error in (no error)"=w6419, "Interface in"=w6421) -> ("error out"=w6417:errorcluster, "prev ExpTime"=w6414:dbl, "Interface out"=w6415:refnum<class "Interface.lvclass">)  [unwired: 7 in]
                n2857 = property on="Exptime ch2" class="DigNum (strict)"(error in=w6417, "Value"=w6414) -> (error out=w6416:errorcluster)  [unwired: 1 in, 1 out]
                n2858 = call "Write Exposure Time.vi"("error in (no error)"=w6416, "Exposure Time"=w6414, "Interface in"=w6415) -> ("error out"=w6413:errorcluster, "Interface out"=w6412:refnum<class "Interface.lvclass">)  [unwired: 7 in]
              }
            }
            n2859 = case shown="True" w6199 {
              tunnel: [w6424 w6425] -> w6205
              tunnel: [w6423 w6426] -> w6204
              tunnel: w6201 -> [w6424 w6435]
              tunnel: w6200 -> [w6423 w6433]
              frame False {
              }
              frame True {
                n2860 = call-dynamic "Write restoreExpTime.vi"("error in (no error)"=w6433, "restoreExpTime"=FALSE, "Interface in"=w6435) -> ("error out"=w6432:errorcluster, "Interface out"=w6434:refnum<class "Interface.lvclass">)  [unwired: 7 in]
                n2861 = call-dynamic "Read prev ExpTime.vi"("error in (no error)"=w6432, "Interface in"=w6434) -> ("error out"=w6428:errorcluster, "prev ExpTime"=w6429:dbl, "Interface out"=w6430:refnum<class "Interface.lvclass">)  [unwired: 7 in]
                n2862 = property on="Exptime ch1" class="DigNum (strict)"(error in=w6428, "Value"=w6429) -> (error out=w6427:errorcluster)  [unwired: 1 in, 1 out]
                n2863 = call "Write Exposure Time.vi"("error in (no error)"=w6427, "Exposure Time"=w6429, "Interface in"=w6430) -> ("error out"=w6426:errorcluster, "Interface out"=w6425:refnum<class "Interface.lvclass">)  [unwired: 7 in]
              }
            }
            n2864 = call-dynamic "Read PREV_FT.vi"("error in (no error)"=w6046, "Interface in"=w6045) -> ("error out"=w6038:errorcluster, "PREV_FT"=w6047:bool, "Interface out"=w6036:refnum<class "Interface.lvclass">)  [unwired: 7 in]
            n2865 = call-dynamic "Read PREV_FT.vi"("error in (no error)"=w6151, "Interface in"=w6152) -> ("error out"=w6144:errorcluster, "PREV_FT"=w6153:bool, "Interface out"=w6142:refnum<class "Interface.lvclass">)  [unwired: 7 in]
            n2866 = call-dynamic "Read PREV_FT.vi"("error in (no error)"=w6204, "Interface in"=w6205) -> ("error out"=w6195:errorcluster, "PREV_FT"=w6206:bool, "Interface out"=w6190:refnum<class "Interface.lvclass">)  [unwired: 7 in]
            n2867 = call-dynamic "Read PREV_FT.vi"("error in (no error)"=w6098, "Interface in"=w6099) -> ("error out"=w6091:errorcluster, "PREV_FT"=w6100:bool, "Interface out"=w6089:refnum<class "Interface.lvclass">)  [unwired: 7 in]
            n2868 = call-dynamic "Read target cluster.vi"("error in (no error)"=w6038, "Channel in"=w6039) -> ("error out"=w6033:errorcluster, "target cluster"=w6037:T31, "Channel out"=w6035:refnum<class "Channel.lvclass">)  [unwired: 7 in]
            n2869 = Bundle By Name(cluster=w6037, "SHUTTER_MODE"=u8 2, "FRAME_TRANSFER"=w6047) -> (w6034:T31)
            n2870 = call-dynamic "Read target cluster.vi"("error in (no error)"=w6144, "Channel in"=w6145) -> ("error out"=w6139:errorcluster, "target cluster"=w6143:T31, "Channel out"=w6141:refnum<class "Channel.lvclass">)  [unwired: 7 in]
            n2871 = Bundle By Name(cluster=w6143, "SHUTTER_MODE"=u8 2, "FRAME_TRANSFER"=w6153) -> (w6140:T31)
            n2872 = call-dynamic "Read target cluster.vi"("error in (no error)"=w6091, "Channel in"=w6092) -> ("error out"=w6086:errorcluster, "target cluster"=w6090:T31, "Channel out"=w6088:refnum<class "Channel.lvclass">)  [unwired: 7 in]
            n2873 = Bundle By Name(cluster=w6090, "SHUTTER_MODE"=u8 2, "FRAME_TRANSFER"=w6100) -> (w6087:T31)
            n2874 = call-dynamic "Read target cluster.vi"("error in (no error)"=w6195, "Channel in"=w6198) -> ("error out"=w6194:errorcluster, "target cluster"=w6192:T31, "Channel out"=w6197:refnum<class "Channel.lvclass">)  [unwired: 7 in]
            n2875 = Bundle By Name(cluster=w6192, "SHUTTER_MODE"=u8 2, "FRAME_TRANSFER"=w6206) -> (w6191:T31)
            n2876 = call-dynamic "Write target cluster.vi"("error in (no error)"=w6194, "target cluster"=w6191, "Channel in"=w6197) -> ("error out"=w6193:errorcluster, "Channel out"=w6196:refnum<class "Channel.lvclass">)  [unwired: 7 in]
            n2877 = call-dynamic "Write target cluster.vi"("error in (no error)"=w6033, "target cluster"=w6034, "Channel in"=w6035) -> ("error out"=w6032:errorcluster, "Channel out"=w6031:refnum<class "Channel.lvclass">)  [unwired: 7 in]
            n2878 = call-dynamic "Write target cluster.vi"("error in (no error)"=w6139, "target cluster"=w6140, "Channel in"=w6141) -> ("error out"=w6138:errorcluster, "Channel out"=w6137:refnum<class "Channel.lvclass">)  [unwired: 7 in]
            n2879 = call-dynamic "Write target cluster.vi"("error in (no error)"=w6086, "target cluster"=w6087, "Channel in"=w6088) -> ("error out"=w6085:errorcluster, "Channel out"=w6084:refnum<class "Channel.lvclass">)  [unwired: 7 in]
            n2880 = Flatten To String(anything=w6191, error in (no error)=w6193) -> (data string=w6239:string, error out=w6238:errorcluster)  [unwired: 2 in, 1 out]
